vi "TPNT_GetDeviceHelp.vi"(10 "name":string) -> (2 "help":string)   [LabVIEW 2016]
uses:
  TPNT_DeviceTPs.ctl
  TPNT_TP.ctl
  TPNT_Limits.ctl
  TPNT_Samples.ctl
  TPNT_Log.ctl
panel:
  in  "TPNT_DeviceTPs":T1={"device"="", "devupdate"=0.0, "next_update"=0, "devinterface"="", "TPs"=[], "Alarms"=TRUE, "monitor"=TRUE, "log sep"=""} {"TPs"."Log"."updaterate" format="%.2f"; "TPs"."Samples"."Values" format="%.2f"; "TPs"."Samples"."samples" min=1 step=1; "TPs"."Limits"."Nominal" format="%.2f"; "TPs"."Limits"."Upper" format="%.2f"; "TPs"."Limits"."Lower" format="%.2f"; "TPs"."update_rate" format="%.2f"; "devupdate" format="%.2f"}
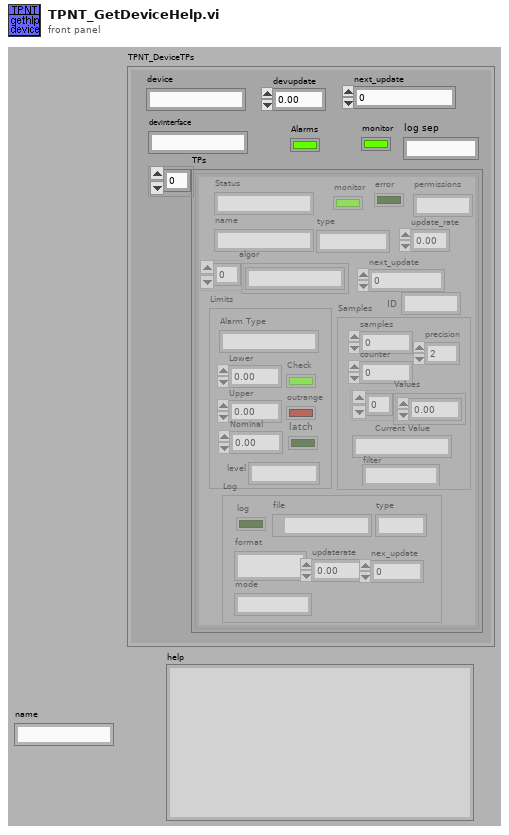
[diagram p1: front panel]
types:
  T1 = typedef "TPNT_DeviceTPs.ctl" = cluster{"device":string, "devupdate":dbl, "next_update":u32, "devinterface":string, "TPs":T2[], "Alarms":bool, "monitor":bool, "log sep":string}
  T2 = typedef "TPNT_TP.ctl" = cluster{"name":string, "type":string, "algor":string[], "update_rate":sgl, "Limits":T3, "Samples":T4, "next_update":u32, "Status":string, "monitor":bool, "error":bool, "Log":T5, "permissions":string, "ID":string}
  T3 = typedef "TPNT_Limits.ctl" = cluster{"Alarm Type":string, "Lower ":dbl, "Upper":dbl, "Nominal":dbl, "outrange":bool, "Check":bool, "latch":bool, "level":string}
  T4 = typedef "TPNT_Samples.ctl" = cluster{"samples":i32, "counter":i32, "Values":dbl[], "Current Value":string, "filter":string, "precision":u8}
  T5 = typedef "TPNT_Log.ctl" = cluster{"log":bool, "file":path, "type":string, "format":string, "updaterate":dbl, "nex_update":u32, "mode":string}
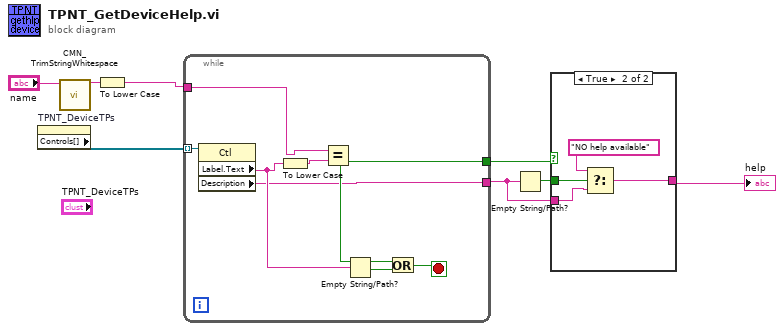
[diagram p0: block diagram]
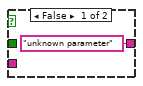
[diagram p2: hidden frame]
diagram:
  n1 = property on="TPNT_DeviceTPs" class="Clust (strict)"() -> ("Controls[]"=w3:refnum<vi>[])  [unwired: 2 in, 2 out]
  n2 = call "CMN_TrimStringWhitespace.vi"("string"="name") -> ("trimmed string"=w1:string)  [unwired: 1 in, 8 out]
  n3 = To Lower Case(string=w1) -> (all lower case string=w8:string)
  n4 = while {
    tunnel: w3 -> [w16] mode=indexing
    tunnel: w8 -> [w13]
    tunnel: [w10] -> w7
    tunnel: [w9] -> w4
    stop <- w14 stop-if-true
    n5 = property class="Ctl"(reference=w16) -> ("Label.Text"=w12:string, "Description"=w9:string)  [unwired: 1 in, 2 out]
    n6 = To Lower Case(string=w12) -> (all lower case string=w11:string)
    n7 = Equal?(x=w13, y=w11) -> (x = y?=w10:bool)
    n8 = Empty String/Path?(string/path=w12) -> (empty?=w15:bool)
    n9 = Or(x=w10, y=w15) -> (x .or. y?=w14:bool)
  }
  n10 = Empty String/Path?(string/path=w4) -> (empty?=w5:bool)
  n11 = case shown="True" w7 {
    tunnel: ["unknown parameter" ("Desc") w19] -> w6
    tunnel: w5 -> [_ w21]
    tunnel: w4 -> [_ w20]
    frame False {
    }
    frame True {
      n12 = Select(t="NO help available", s=w21, f=w20) -> (s? t:f=w19:string)
    }
  }
  "help" <- w6
